vi "AI Configurations.vi"(2 "Auto control  max AI rate/ AI block size":bool=TRUE, 3 "Max AI Rate In":i32=10000, 4 "Frequency In":dbl) -> (0 "AI Rate Out":i32, 1 "AI Block Size Out":dbl)   [LabVIEW 2013, in "Lock-In Variable Channels_2.lvclass"]
uses:
  Lock-In Variable Channels_2.lvclass
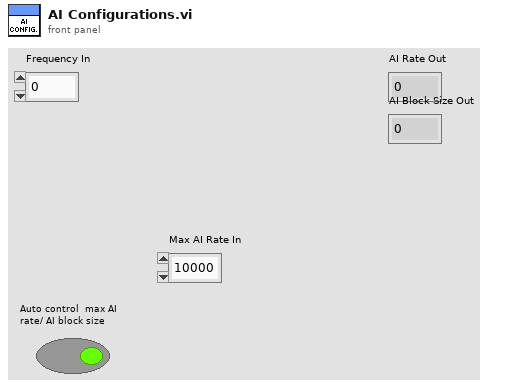
[diagram p1: front panel]
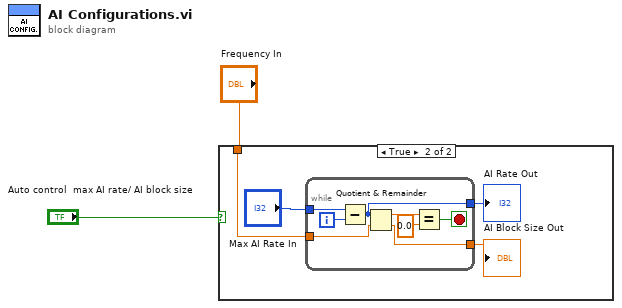
[diagram p0: block diagram]
diagram:
  n1 = case shown="True" "Auto control  max AI rate/ AI block size" {
    tunnel: "Frequency In" -> [_ w5]
    frame False {
    }
    frame True {
      n2 = while {
        tunnel: "Max AI Rate In" -> [w14]
        tunnel: w5 -> [w12]
        tunnel: [w8] -> w3
        tunnel: [w7] -> w4
        i -> [w13]
        stop <- w9 stop-if-true
        n3 = Subtract(x=w14, y=w13) -> (x-y=w7:i32)
        n4 = Quotient & Remainder(x=w7, y=w12) -> (x-y*floor(x/y)=w11:dbl, floor(x/y)=w8:dbl)
        n5 = Equal?(x=w11, y=0.0) -> (x = y?=w9:bool)
      }
      "AI Rate Out" <- w4
      "AI Block Size Out" <- w3
    }
  }
